vi "Drive Async Framework.vi"   [LabVIEW 2015]
doc: "This VI provides a framework for calling drive tasks asynchronously."
uses:
  Robot Global Data.vi
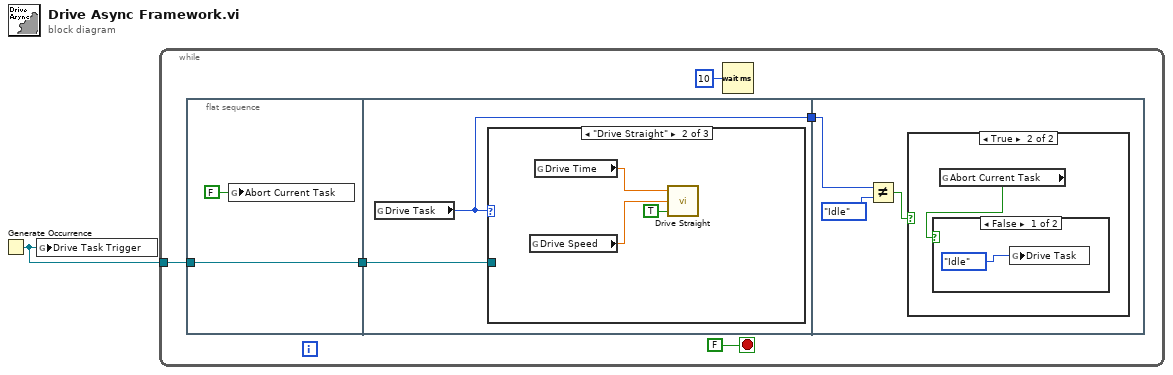
[diagram p0: block diagram]
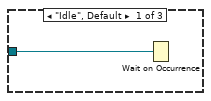
[diagram p2: hidden frame]
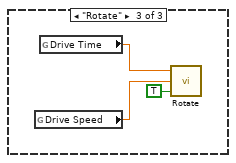
[diagram p3: hidden frame]
diagram:
  n1 = Generate Occurrence() -> (w1:refnum<k4>)
  n2 = global write "Robot Global Data.vi" "Drive Task Trigger"(w1) -> ()
  n3 = while {
    tunnel: w1 -> [w4]
    stop <- FALSE stop-if-true
    n4 = flat-sequence {
      tunnel: w4 -> [w8]
      tunnel: [w8] -> w3
      tunnel: w3 -> [w10]
      tunnel: [w9] -> w2
      tunnel: w2 -> [w20]
      frame #0 {
        n5 = global write "Robot Global Data.vi" "Abort Current Task"(FALSE ("Abort Current Task")) -> ()
      }
      frame #1 {
        n6 = global read "Robot Global Data.vi" "Drive Task"() -> (w9:enum16{"Idle", "Drive Straight", "Rotate"})
        n7 = case shown="\"Drive Straight\"" w9 {
          tunnel: w10 -> [w11 _ _]
          frame "Idle", Default {
            n8 = Wait on Occurrence(2:w11) -> ()  [unwired: 2 in, 1 out]
          }
          frame "Drive Straight" {
            n9 = global read "Robot Global Data.vi" "Drive Speed"() -> (w13:dbl)
            n10 = global read "Robot Global Data.vi" "Drive Time"() -> (w14:dbl)
            n11 = call "Drive Straight.vi"("Asynchronous"=TRUE, "Drive Speed"=w13, "Drive Time"=w14) -> ()  [unwired: 1 in]
          }
          frame "Rotate" {
            n12 = global read "Robot Global Data.vi" "Drive Speed"() -> (w16:dbl)
            n13 = global read "Robot Global Data.vi" "Drive Time"() -> (w17:dbl)
            n14 = call "Rotate.vi"("Asynchronous"=TRUE, "Drive Speed"=w16, "Drive Time"=w17) -> ()  [unwired: 1 in]
          }
        }
      }
      frame #2 {
        n15 = Not Equal?(x=w20, y=enum16{"Idle", "Drive Straight", "Rotate"}."Idle") -> (x != y?=w19:bool)
        n16 = case shown="True" w19 {
          frame False {
          }
          frame True {
            n17 = global read "Robot Global Data.vi" "Abort Current Task"() -> (w21:bool)
            n18 = case shown="False" w21 {
              frame False {
                n19 = global write "Robot Global Data.vi" "Drive Task"(enum16{"Idle", "Drive Straight", "Rotate"}."Idle" ("y")) -> ()
              }
              frame True {
              }
            }
          }
        }
      }
    }
    n20 = Wait (ms)(milliseconds to wait=u32 10) -> ()  [unwired: 1 out]
  }
